vi "Read Hardware Notifier.vi"(8 "error in (no error)":errorcluster, 11 "MFC in":refnum<class "Scale.lvclass">) -> (0 "error out":errorcluster, 2 "Hardware Notifier":refnum<notifier>, 3 "MFC out":refnum<class "Scale.lvclass">)   [LabVIEW 2013, in "Scale.lvlib" / "Scale.lvclass"]
uses:
  Scale.lvclass
  <vilib>/ActorFramework/Time-Delayed Send Message/Time-Delay Override Options.ctl
  Scale.lvclass/Scale.ctl
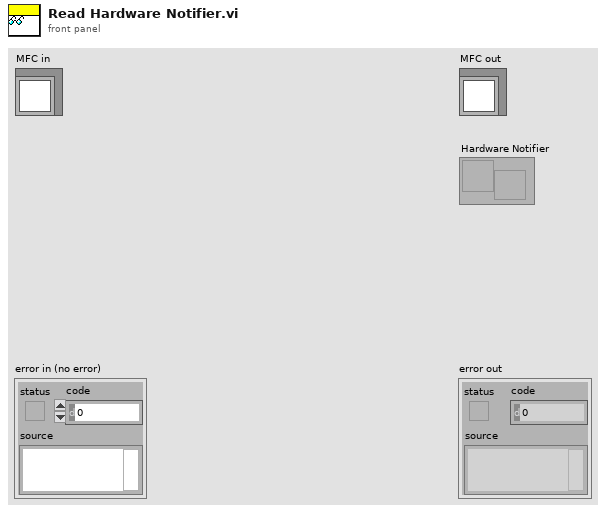
[diagram p1: front panel]
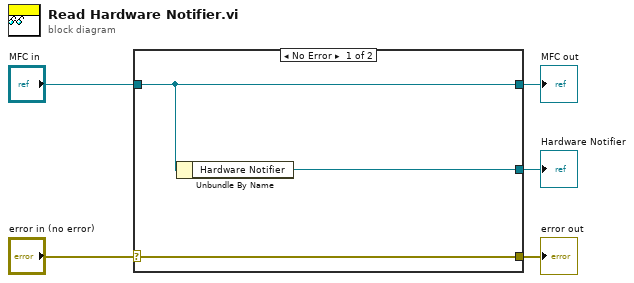
[diagram p0: block diagram]
diagram:
  n1 = case shown="No Error" "error in (no error)" {
    selector: "error in (no error)" -> [w8 w9]
    tunnel: [w8 w9] -> w4
    tunnel: [w7 w10] -> w2
    tunnel: "MFC in" -> [w7 w10]
    tunnel: [w6 _] -> w1
    frame No Error {
      n2 = Unbundle By Name(w7) -> ("Hardware Notifier"=w6:refnum<notifier>)
    }
    frame Error {
    }
  }
  "error out" <- w4
  "MFC out" <- w2
  "Hardware Notifier" <- w1
